vi "Close Log File.vi"(8 "error in (no error)":errorcluster, 11 "Datalogger Actor in":refnum<class "Datalogger Actor.lvclass">) -> (0 "error out":errorcluster, 3 "Datalogger Actor out":refnum<class "Datalogger Actor.lvclass">)   [LabVIEW 2018, in "Datalogger Actor.lvlib" / "Datalogger Actor.lvclass"]
uses:
  Datalogger Actor.lvclass
  Datalogger Actor.lvclass/Datalogger Actor.ctl
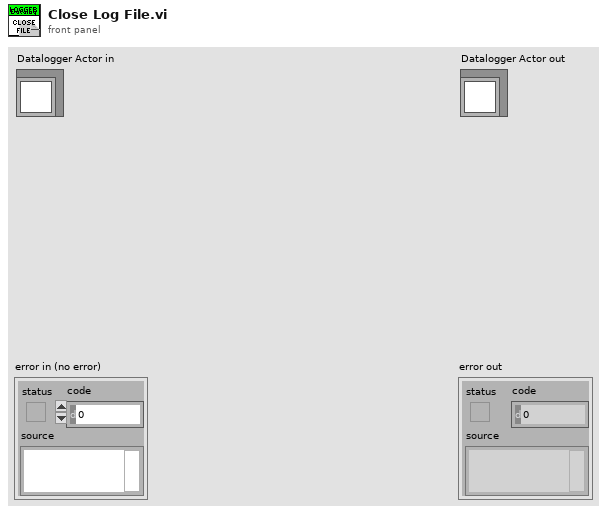
[diagram p1: front panel]
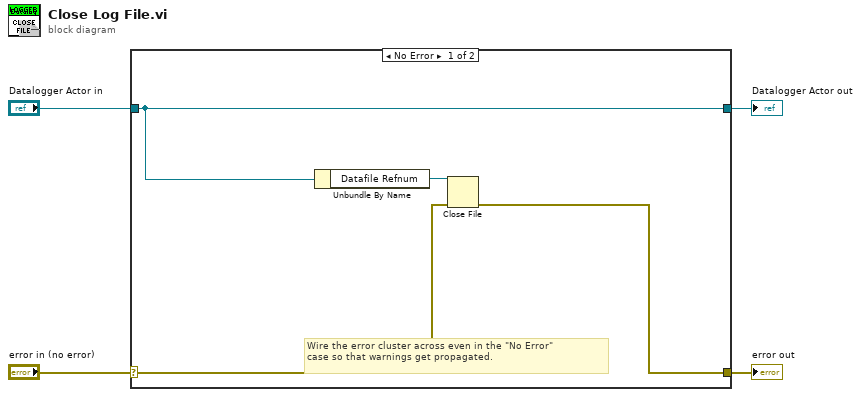
[diagram p0: block diagram]
diagram:
  n1 = case shown="No Error" "error in (no error)" {
    selector: "error in (no error)" -> [w6 w10]
    tunnel: [w5 w10] -> w3
    tunnel: [w8 w9] -> w1
    tunnel: "Datalogger Actor in" -> [w8 w9]
    frame No Error {
      # "Wire the error cluster across even in the \"No Error\"\ncase so that warnings get propagated."
      n2 = Unbundle By Name(w8) -> ("Datafile Refnum"=w7:refnum<file>)
      n3 = Close File(refnum=w7, error in=w6) -> (error out=w5:errorcluster)  [unwired: 1 out]
    }
    frame Error {
    }
  }
  "error out" <- w3
  "Datalogger Actor out" <- w1
